vi "Choose entry.vi"(1 "Array of strings.":string[](array[string]), 2 "Selection start.":sgl format="%.2f", 3 "Array of string lengths.":sgl[](array[numeric]) format="%.2f") -> (0 "Selected string.":string)   [LabVIEW 2010]
panel:
  # "Outputs:"
  # "Inputs:"
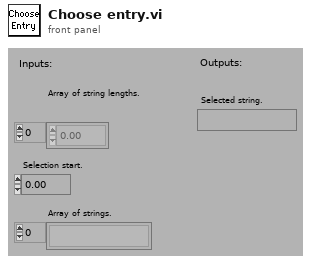
[diagram p1: front panel]
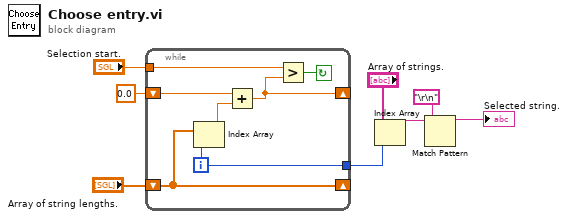
[diagram p0: block diagram]
diagram:
  n1 = while {
    tunnel: [w14] -> w7
    tunnel: "Selection start." -> [w11]
    shift-left: sgl 0.0 -> [w12]
    shift-right: [w10] -> _
    shift-left: "Array of string lengths." -> [w15]
    shift-right: [w15] -> _
    i -> [w14]
    stop <- w9 continue-if-true
    n2 = Index Array(array=w15, index=w14) -> (element=w13:sgl)
    n3 = Add(x=w12, y=w13) -> (x+y=w10:sgl)
    n4 = Greater?(x=w11, y=w10) -> (0:w9:bool)
  }
  n5 = Index Array(array="Array of strings.", index=w7) -> (element=w5:string)
  n6 = Match Pattern(string=w5, regular expression="\r\n") -> (before substring=→"Selected string.":string)  [unwired: 4 out]
